vi "Prasing Frame.vi"(8 "error in (no error)":errorcluster caption="entrée d'erreur (pas d'erreur)", 11 "Class UART Nodon.lvclass En entrée":refnum<class "Class UART Nodon.lvclass">) -> (0 "error out":errorcluster caption="sortie d'erreur", 3 "Class UART Nodon.lvclass En sortie":refnum<class "Class UART Nodon.lvclass">)   [LabVIEW 2020, in "Library Instrument & Equipement.lvlib" / "Library UART.lvlib" / "Class UART Nodon.lvclass"]
uses:
  Class UART Nodon.lvclass
  C:/Users/ngarcin/OneDrive - Altyor/Standard TB/Class/UART/UART (Default)/Class UART (Default).lvclass
  Class UART Nodon.lvclass/Class UART Nodon.ctl
  Commun VI/Library Commun.lvlib
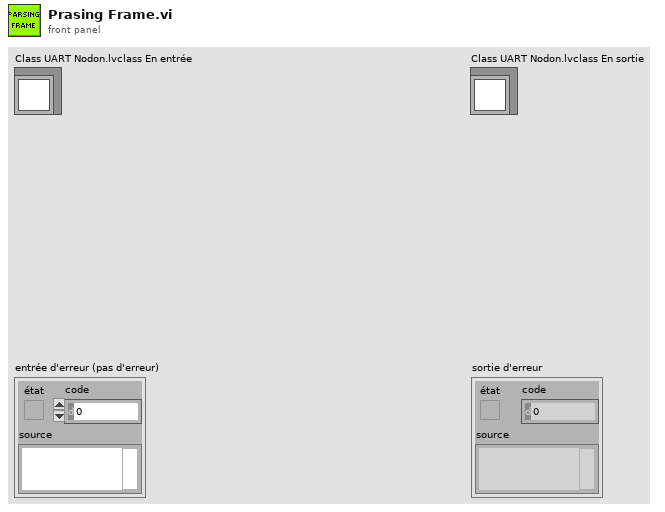
[diagram p1: front panel]
types:
  T1 = enum16{"Wait Data Start", "Wait Lenght", "Check Frame", "Wait Size Data"}[]
  T2 = enum16{"CRC Altyor", "CRC Xor On all Bytes", "CRC8", "CRC16", "CRC32", "Other"}
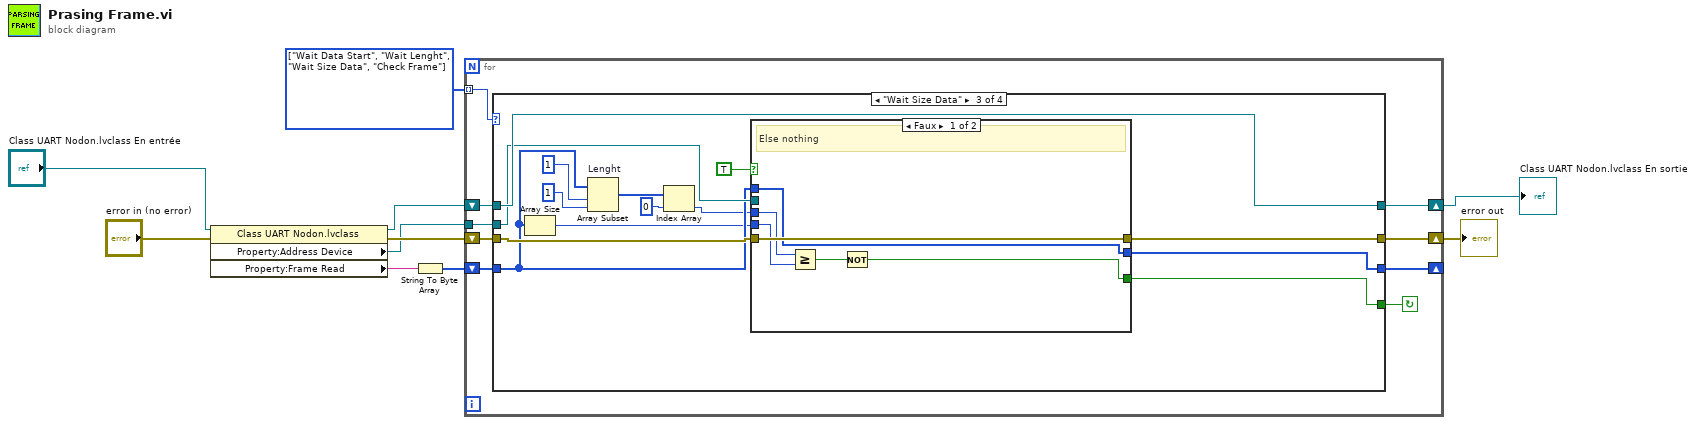
[diagram p0: block diagram]
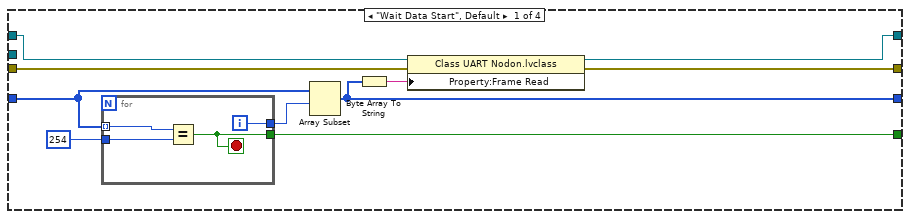
[diagram p2: hidden frame]
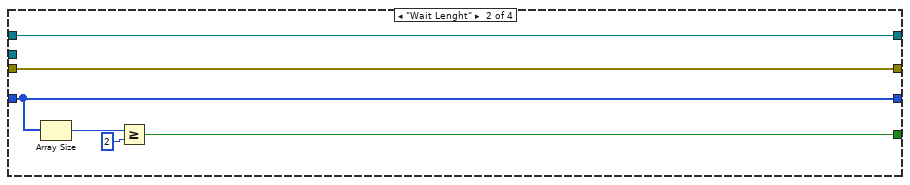
[diagram p3: hidden frame]
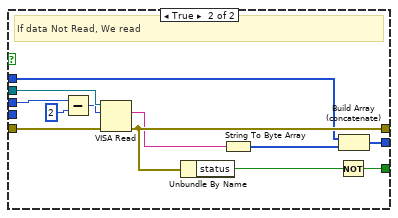
[diagram p4: hidden frame]
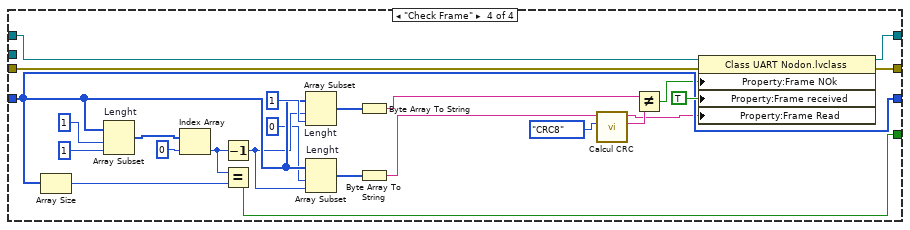
[diagram p5: hidden frame]
diagram:
  w8 = T1 [enum."Wait Data Start", enum."Wait Lenght", enum."Wait Size Data", enum."Check Frame"] items=["Wait Data Start", "Wait Lenght", "Check Frame", "Wait Size Data"]
  n1 = property class="Class UART Nodon.lvclass"(reference="Class UART Nodon.lvclass En entrée", error in="error in (no error)") -> (reference out=w6:refnum<class "Class UART Nodon.lvclass">, error out=w3:errorcluster, "Property:Address Device"=w1:refnum<visa-resource-name>, "Property:Frame Read"=w2:string)
  n2 = String To Byte Array(string=w2) -> (unsigned byte array=w7:u8[])
  n3 = for {
    tunnel: w8 -> [w18] mode=indexing
    shift-right: [w15] -> w5
    shift-left: w6 -> [w16]
    shift-right: [w13] -> w4
    shift-left: w3 -> [w14]
    shift-right: [w12] -> _
    shift-left: w7 -> [w19]
    tunnel: w1 -> [w11]
    stop <- w17 continue-if-true
    n4 = case shown="\"Wait Size Data\"" w18 {
      tunnel: w19 -> [w23 w39 w43 w82]
      tunnel: [w28 w36 w45 w87] -> w17
      tunnel: w16 -> [w27 w35 w53 w94]
      tunnel: [w26 w35 w53 w91] -> w15
      tunnel: w14 -> [w25 w34 w48 w93]
      tunnel: [w24 w34 w46 w92] -> w13
      tunnel: [w20 w39 w44 w82] -> w12
      tunnel: w11 -> [_ _ w47 _]
      frame "Wait Data Start", Default {
        n5 = for {
          tunnel: w23 -> [w33] mode=indexing
          tunnel: [w32] -> w22
          tunnel: u8 254 -> [w31]
          tunnel: [w30] -> w28
          i -> [w32]
          stop <- w30 stop-if-true
          n6 = Equal?(x=w33, y=w31) -> (x = y?=w30:bool)
        }
        n7 = Array Subset(array=w23, index=w22) -> (w20:u8[])  [unwired: 1 in]
        n8 = Byte Array To String(unsigned byte array=w20) -> (string=w21:string)
        n9 = property class="Class UART Nodon.lvclass"(reference=w27, error in=w25, "Property:Frame Read"=w21) -> (reference out=w26:refnum<class "Class UART Nodon.lvclass">, error out=w24:errorcluster)
      }
      frame "Wait Lenght" {
        n10 = Array Size(array=w39) -> (size(s)=w38:i32)
        n11 = Greater Or Equal?(x=w38, y=2) -> (x >= y?=w36:bool)
      }
      frame "Wait Size Data" {
        n12 = Array Size(array=w43) -> (size(s)=w41:i32)
        n13 = Array Subset "Lenght"(array=w43, index=1 ("indice"), length=1 ("longueur")) -> (w50:u8[])
        n14 = Index Array(array=w50, index=0 ("indice")) -> (element=w40:u8)
        n15 = case shown="Faux" TRUE {
          tunnel: w48 -> [w59 w71]
          tunnel: w47 -> [_ w70]
          tunnel: [w59 w69] -> w46
          tunnel: [w57 w67] -> w45
          tunnel: [w58 w64] -> w44
          tunnel: w43 -> [w58 w63]
          tunnel: w40 -> [w54 w62]
          tunnel: w41 -> [w56 _]
          frame False {
            # "Else nothing"
            n16 = Greater Or Equal?(x=w54, y=w56) -> (x >= y?=w55:bool)
            n17 = Not(x=w55) -> (.not. x?=w57:bool)
          }
          frame True {
            # "If data Not Read, We read"
            n18 = Subtract(x=w62, y=u8 2) -> (x-y=w60:u8)
            n19 = VISA Read(VISA resource name=w70, byte count=w60, error in (no error)=w71) -> (read buffer=w66:string, error out=w69:errorcluster)  [unwired: 2 out]
            n20 = Unbundle By Name(w69) -> ("status"=w68:bool)
            n21 = String To Byte Array(string=w66) -> (unsigned byte array=w65:u8[])
            n22 = Not(x=w68) -> (.not. x?=w67:bool)
            n23 = Build Array (concatenate)(w63, w65) -> (w64:u8[])
          }
        }
      }
      frame "Check Frame" {
        n24 = Array Size(array=w82) -> (size(s)=w88:i32)
        n25 = Array Subset "Lenght"(array=w82, index=1 ("indice"), length=1 ("longueur")) -> (w90:u8[])
        n26 = Index Array(array=w90, index=0 ("indice")) -> (element=w83:u8)
        n27 = Decrement(x=w83) -> (x-1=w81:u8)
        n28 = Equal?(x=w83, y=w88) -> (x = y?=w87:bool)
        n29 = Array Subset "Lenght"(array=w82, index=w81, length=1 ("longueur")) -> (w76:u8[])
        n30 = Array Subset "Lenght"(array=w82, index=0 ("indice"), length=w81) -> (w79:u8[])
        n31 = Byte Array To String(unsigned byte array=w76) -> (string=w75:string)
        n32 = Byte Array To String(unsigned byte array=w79) -> (string=w78:string)
        n33 = call "Calcul CRC.vi"("CRC type"=T2."CRC8", "Trame"=w78) -> ("CRC"=w77:string, "Trame + CRC"=w72:string)  [unwired: 8 in]
        n34 = Not Equal?(x=w75, y=w77) -> (x != y?=w74:bool)
        n35 = property class="Class UART Nodon.lvclass"(reference=w94, error in=w93, "Property:Frame NOk"=w74, "Property:Frame received"=TRUE ("Frame received"), "Property:Frame Read"=w72) -> (reference out=w91:refnum<class "Class UART Nodon.lvclass">, error out=w92:errorcluster)
      }
    }
  }
  "error out" <- w4
  "Class UART Nodon.lvclass En sortie" <- w5
